vi "sys class.vi"(8 "error in (no error)":errorcluster caption="错误输入（无错误）", 11 "应用程序输入":refnum<vi>) -> (0 "error out":errorcluster caption="错误输出", 3 "Development System？":bool)   [LabVIEW 2018]
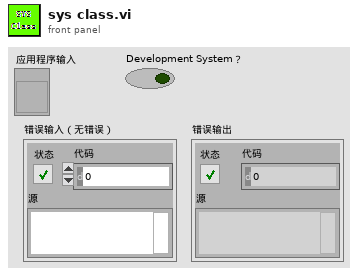
[diagram p1: front panel]
types:
  T1 = enum32{"invalid app kind", "Development System", "Run Time System", "Student Edition", "Embedded LabVIEW", "Evaluation", "Custom"}
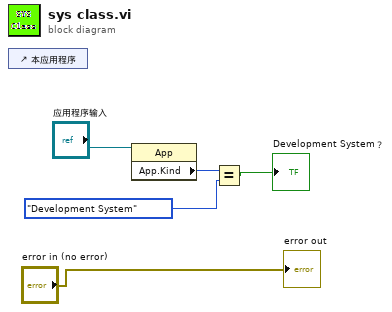
[diagram p0: block diagram]
diagram:
  n1 = control-ref of="本应用程序"() -> ()  [unwired: 1 out]
  n2 = property class="App"(reference="应用程序输入") -> ("App.Kind"=w3:T1)  [unwired: 1 in, 2 out]
  n3 = Equal?(x=w3, y=T1."Development System" ("应用程序:类别")) -> (x = y?=→"Development System？":bool)
  "error out" <- "error in (no error)"
